vi "ad2deg.vi"(2 "DEC (sec)":dbl format="%<%H:%M:%S%1u>t", 3 "RA (sec)":dbl format="%<%H:%M:%S%2u>t") -> (0 "DEC (°)":dbl format="%.8g", 1 "RA (°)":dbl format="%.8g")   [LabVIEW 2011]
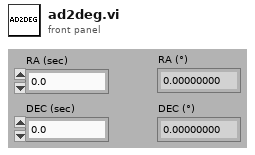
[diagram p1: front panel]
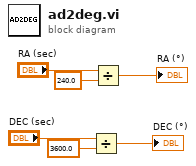
[diagram p0: block diagram]
diagram:
  n1 = Divide(x="DEC (sec)", y=3600.0) -> (x/y=→"DEC (°)":dbl)
  n2 = Divide(x="RA (sec)", y=240.0) -> (x/y=→"RA (°)":dbl)
